vi "ScaleVision.vi"(7 "Save":bool, 8 "error in":errorcluster, 9 "CopyImageRef":T2, 10 "VisionImageRef":T2, 11 "CameraSession":T1) -> (0 "error out":errorcluster, 1 "VisionLoopRate":dbl, 2 "Image":T2(plugin-control), 3 "ScaleAngleDegrees":dbl)   [LabVIEW 2017]
uses:
  <vilib>/vision/Image Controls.llb/IMAQ Image.ctl
  <vilib>/userdefined/High Color/IMAQdx.ctl
  <vilib>/vision/driver/NI_Vision_Acquisition_Software.lvlib
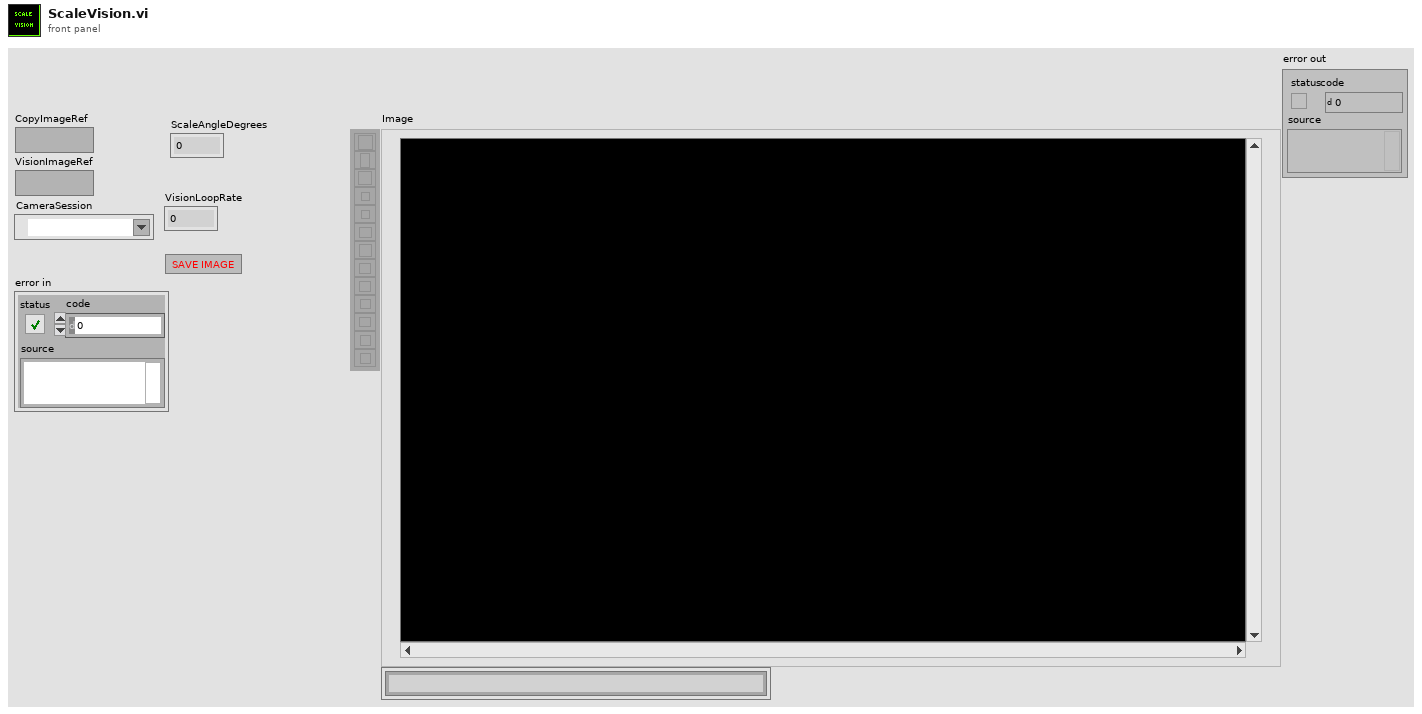
[diagram p1: front panel]
types:
  T1 = typedef "IMAQdx.ctl" = refnum<k21>
  T2 = typedef "IMAQ Image.ctl" = refnum<image>
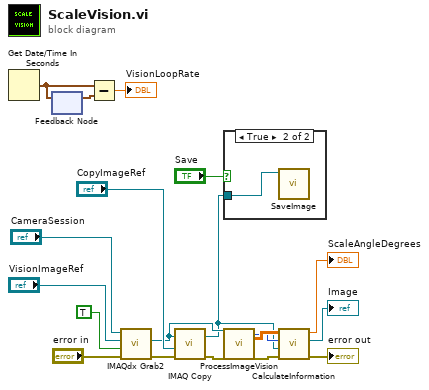
[diagram p0: block diagram]
diagram:
  n1 = Get Date/Time In Seconds() -> (seconds since 1Jan1904=w15:timestamp)
  n2 = feedback #1() -> (w14:timestamp)  [unwired: 1 in]
  n3 = feedback-in #1(w15) -> ()
  n4 = Subtract(x=w15, y=w14) -> (x-y=→"VisionLoopRate":dbl)
  n5 = call <vilib>:"IMAQdx Grab2.vi"("error in"="error in", "Wait for Next Buffer? (Yes)"=TRUE, "Image In"="VisionImageRef", "Session In"="CameraSession") -> ("error out"=w6:errorcluster, "Image Out"=w11:T2)  [unwired: 4 in, 2 out]
  n6 = call "IMAQ Copy"("error in (no error)"=w6, "Image Dst"="CopyImageRef", "Image Src"=w11) -> ("error out"=w5:errorcluster, "Image Dst Out"=w3:T2)  [unwired: 3 in]
  n7 = case shown="True" "Save" {
    tunnel: w3 -> [_ w20]
    frame False {
    }
    frame True {
      n8 = call "SaveImage.vi"("Refnum in"=w20) -> ()  [unwired: 11 in]
    }
  }
  n9 = call "ProcessImageVision.vi"("Image In"=w11, "error in"=w5) -> ("Number of Particles (Particle Analysis 1)"=w8:i32, "Particle Measurements (Pixels) (Particle Analysis 1)"=w9:dbl[][], "error out"=w4:errorcluster)  [unwired: 22 in, 1 out]
  n10 = call "CalculateInformation.vi"("error in"=w4, "ImageIn"=w3, "Number of Particles"=w8, "Particle Measurements"=w9) -> ("error out"=→"error out":errorcluster, "OverlayImageOut"=→"Image":T2, "ScaleAngleDegrees"=→"ScaleAngleDegrees":dbl)  [unwired: 4 in, 1 out]
